vi "set_origin.vi"(8 "error in (no error)":errorcluster, 11 "StageMH100301DMC in":refnum<class "StageMH100301DMC.lvclass">) -> (0 "error out":errorcluster, 3 "StageMH100301DMC out":refnum<class "StageMH100301DMC.lvclass">)   [LabVIEW 2010, in "StageMH100301DMC.lvclass"]
uses:
  StageMH100301DMC.lvclass
  StageDL090409Scaffold/StageDL090409Scaffold/StageDL090409Scaffold.lvclass
  common/classes/ErrorController/ErrorController/class_data.vi
  common/classes/ErrorController/ErrorController/ErrorController.lvclass
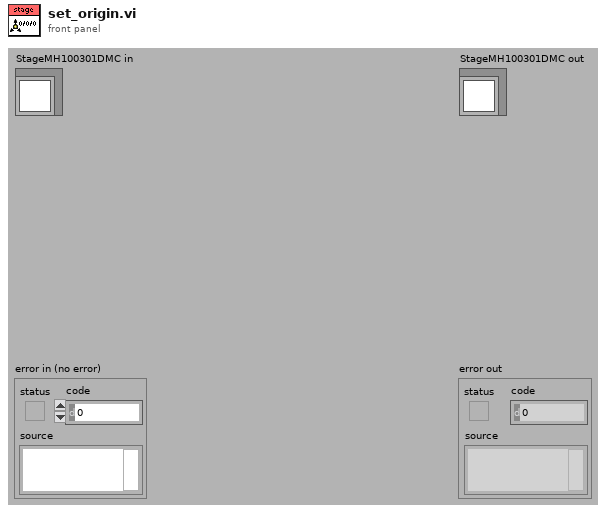
[diagram p1: front panel]
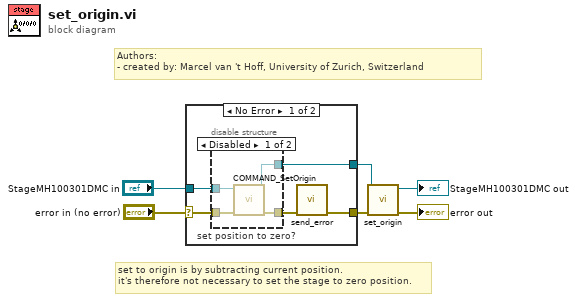
[diagram p0: block diagram]
diagram:
  # "set to origin is by subtracting current position.\nit's therefore not necessary to set the stage to zero position."
  # "Authors: \n- created by: Marcel van 't Hoff, University of Zurich, Switzerland"
  n1 = case shown="No Error" "error in (no error)" {
    selector: "error in (no error)" -> [w10 w18]
    tunnel: [w9 w18] -> w2
    tunnel: [w8 w19] -> w1
    tunnel: "StageMH100301DMC in" -> [w11 w19]
    frame No Error {
      n2 = disable-structure "set position to zero?" shown="Disabled" {
        disable-tunnel: w11 -> [w15 w17]
        disable-tunnel: w10 -> [w14 w16]
        disable-tunnel: [w13 w17] -> w8
        disable-tunnel: [w12 w16] -> w7
        frame Disabled {
          n3 = call-dynamic "COMMAND_SetOrigin.vi"("error in (no error)"=w14, "MH100301DMC in"=w15) -> ("error out"=w12:errorcluster, "MH100301DMC out"=w13:refnum<class "StageMH100301DMC.lvclass">)  [unwired: 8 in]
        }
        frame Enabled {
        }
      }
      n4 = call "send_error.vi"("error in (no error)"=w7) -> ("error out"=w9:errorcluster)  [unwired: 10 in]
    }
    frame Error {
    }
  }
  n5 = call-parent "set_origin.vi"("error in (no error)"=w2, "StageDL090409Scaffold in"=w1) -> ("error out"=→"error out":errorcluster, "StageDL090409Scaffold out"=→"StageMH100301DMC out":refnum<class "StageMH100301DMC.lvclass">)  [unwired: 8 in]
